vi "setUp.vi"(8 "error in (no error)":errorcluster, 11 "reference in":refnum<class "TestProtectedSubpanel.lvclass">) -> (0 "error out":errorcluster, 3 "reference out":refnum<class "TestProtectedSubpanel.lvclass">)   [LabVIEW 2015, in "TestProtectedSubpanel.lvclass"]
doc: "setUp runs prior to the test method during test execution. Use this method to initialize any object data required by your tests."
uses:
  TestProtectedSubpanel.lvclass
  Doubles/ViewableDoubles/ViewableOne/ViewableOne.lvclass
  Doubles/ViewableDoubles/ViewableTwo/ViewableTwo.lvclass
  Framework/IViewable/IViewable/IViewable.lvclass
  Doubles/ViewableDoubles/LeakyViewable/LeakyViewable.lvclass/LeakyViewable.ctl
  TestProtectedSubpanel.lvclass/TestProtectedSubpanel.ctl
  <vilib>/addons/_JKI Toolkits/VI Tester/TestCase.llb/TestCase.lvclass
  <vilib>/ActorFramework/Actor/Actor.lvclass
  Doubles/ViewableDoubles/LeakyViewable/LeakyViewable.lvclass
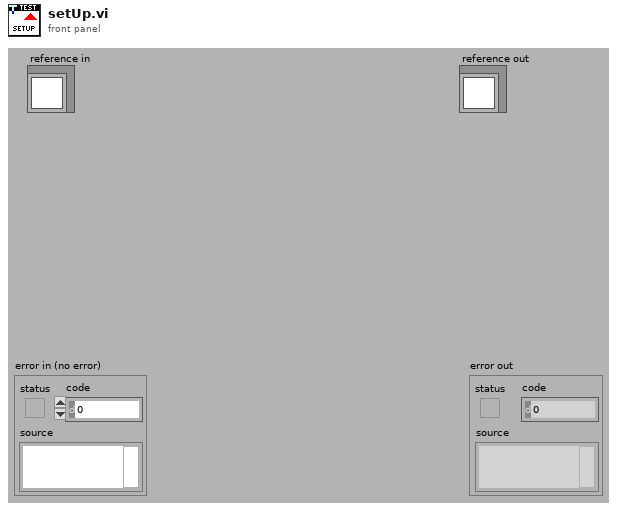
[diagram p1: front panel]
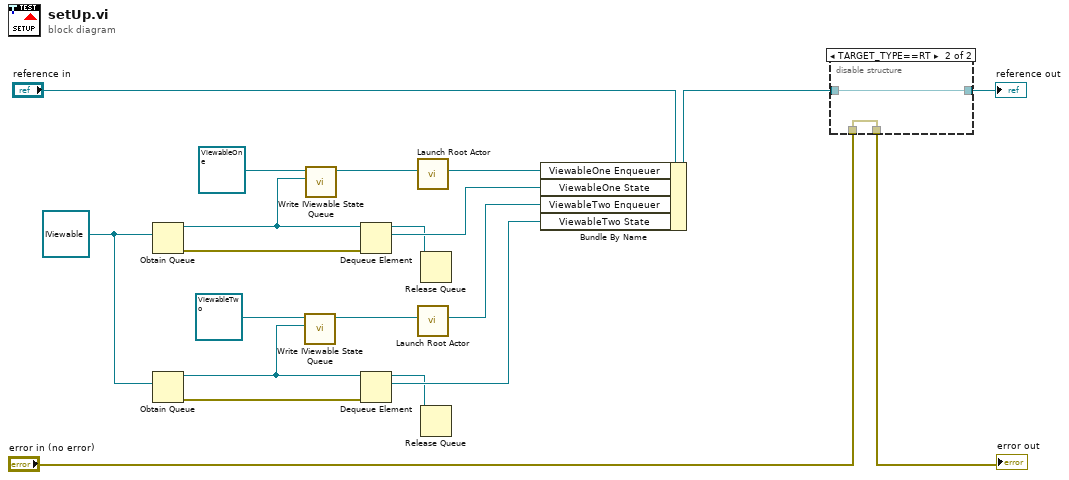
[diagram p0: block diagram]
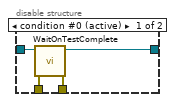
[diagram p2: hidden frame]
diagram:
  w3 = refnum<class "IViewable.lvclass"> refnum ("IViewable.lvlib:IViewable.lvclass")
  n1 = Obtain Queue(element data type=w3) -> (queue out=w8:refnum<queue>, error out=w12:errorcluster)  [unwired: 4 in, 1 out]
  n2 = Obtain Queue(element data type=w3) -> (queue out=w13:refnum<queue>, error out=w11:errorcluster)  [unwired: 4 in, 1 out]
  n3 = call "Write IViewable State Queue.vi"("Viewable State Queue"=w13, "LeakyViewable In"=refnum<class "ViewableTwo.lvclass"> refnum ("ViewableDoubles.lvlib:ViewableTwo.lvclass")) -> ("LeakyViewable Out"=w1:refnum<class "ViewableTwo.lvclass">)  [unwired: 9 in]
  n4 = call "Write IViewable State Queue.vi"("Viewable State Queue"=w8, "LeakyViewable In"=refnum<class "ViewableOne.lvclass"> refnum ("ViewableDoubles.lvlib:ViewableOne.lvclass")) -> ("LeakyViewable Out"=w2:refnum<class "ViewableOne.lvclass">)  [unwired: 9 in]
  n5 = Dequeue Element(queue=w8, error in (no error)=w12) -> (queue out=w5:refnum<queue>, element=w10:refnum<class "IViewable.lvclass">)  [unwired: 1 in, 2 out]
  n6 = Dequeue Element(queue=w13, error in (no error)=w11) -> (queue out=w4:refnum<queue>, element=w9:refnum<class "IViewable.lvclass">)  [unwired: 1 in, 2 out]
  n7 = call <vilib>:"Launch Root Actor.vi"("Actor"=w2) -> ("Actor's Enqueuer"=w7:refnum<class "Message Enqueuer.lvclass">)  [unwired: 9 in, 1 out]
  n8 = call <vilib>:"Launch Root Actor.vi"("Actor"=w1) -> ("Actor's Enqueuer"=w6:refnum<class "Message Enqueuer.lvclass">)  [unwired: 9 in, 1 out]
  n9 = Release Queue(queue=w5) -> ()  [unwired: 2 in, 3 out]
  n10 = Release Queue(queue=w4) -> ()  [unwired: 2 in, 3 out]
  n11 = Bundle By Name(cluster="reference in", "ViewableOne Enqueuer"=w7, "ViewableOne State"=w10, "ViewableTwo Enqueuer"=w6, "ViewableTwo State"=w9) -> (w16:refnum<class "TestProtectedSubpanel.lvclass">)
  n12 = disable-structure shown="TARGET_TYPE==RT" {
    disable-tunnel: "error in (no error)" -> [w24 w25]
    disable-tunnel: [w23 w25] -> w19
    disable-tunnel: [w22 w26] -> w17
    disable-tunnel: w16 -> [w21 w26]
    frame condition #0 (active) {
      n13 = call <vilib>:"WaitOnTestComplete.vi"("error in (no error)"=w24, "TestCase in"=w21) -> ("error out"=w23:errorcluster, "TestCase out"=w22:refnum<class "TestProtectedSubpanel.lvclass">)  [unwired: 8 in]
    }
    frame condition #1 {
    }
  }
  "error out" <- w19
  "reference out" <- w17
